vi "PSTR-Show PSTHs.vi"(0 "Data":T1, 5 "XYGraph":refnum<vi>, 7 "Freq":u16, 9 "Separation":dbl, 11 "Show fits":bool) -> ()   [LabVIEW 2020]
uses:
  Typedefs/PSTR-Data.ctl
  Typedefs/PSTR-Model Fit.ctl
  Typedefs/PSTR-Fit Parameters.ctl
  epl-vi-lib/Utility VIs/Math VIs/LinSpace (x0-dx-npts).vi
panel:
  # "NF x NL x 2 x Npts"
  # "NF x NL x Npts"
  # "NF x NL"
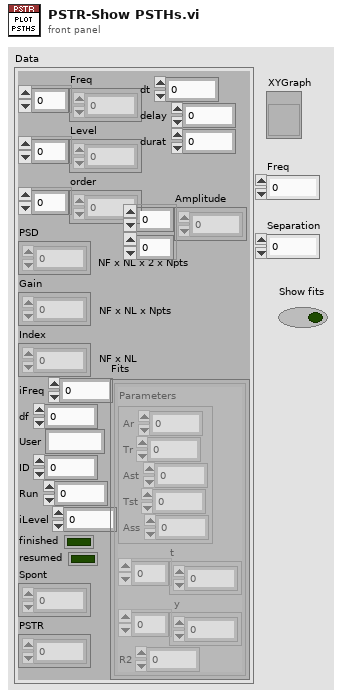
[diagram p1: front panel]
types:
  T1 = typedef "PSTR-Data.ctl" = cluster{"Freq":dbl[], "Level":dbl[], "order":i32[], "PSD":dbl[][][][], "Gain":dbl[][][], "Index":dbl[][], "iFreq":i32, "df":dbl, "User":string, "ID":i32, "Run":i32, "iLevel":i32, "finished":bool, "resumed":bool, "Spont":dbl[][], "PSTR":dbl[][][], "dt":dbl, "delay":dbl, "durat":dbl, "Fits":T2[][], "Amplitude":dbl[][]}
  T2 = typedef "PSTR-Model Fit.ctl" = cluster{"Parameters":T3, "t":dbl[], "y":dbl[], "R2":dbl}
  T3 = typedef "PSTR-Fit Parameters.ctl" = cluster{"Ar":dbl, "Tr":dbl, "Ast":dbl, "Tst":dbl, "Ass":dbl}
  T4 = enum16{"User", "Prism", "Kelly", "Dark2", "Sequential", "Hue"}
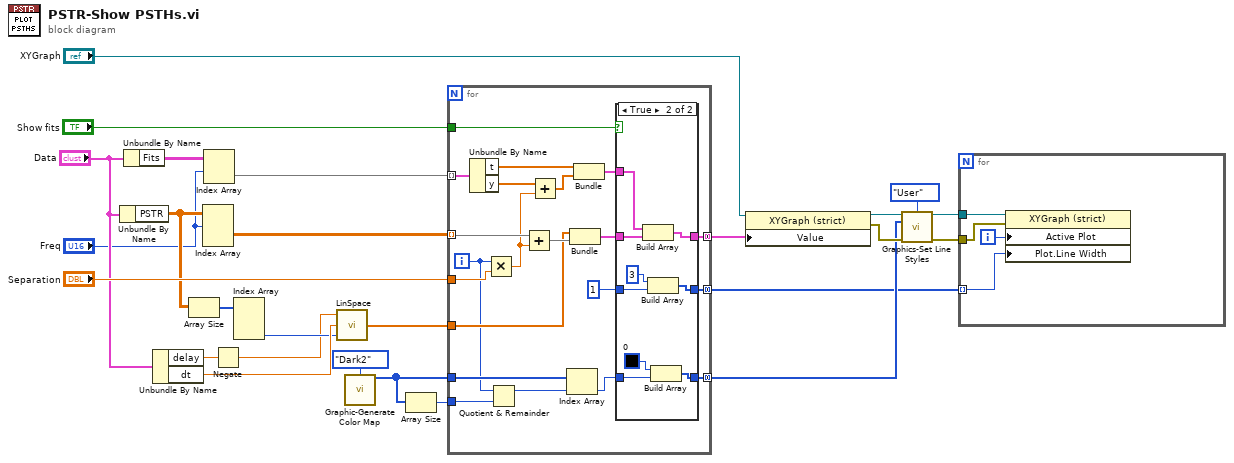
[diagram p0: block diagram]
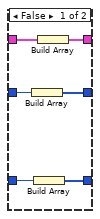
[diagram p2: hidden frame]
diagram:
  n1 = Unbundle By Name("Data") -> ("PSTR"=w21:dbl[][][])
  n2 = Unbundle By Name("Data") -> ("Fits"=w14:T2[][])
  n3 = Unbundle By Name("Data") -> ("delay"=w17:dbl, "dt"=w19:dbl)
  n4 = Array Size(array=w21) -> (size(s)=w20:i32[])
  n5 = Index Array(array=w21, index (dim 0)="Freq") -> (element=w4:dbl[][])  [unwired: 2 in]
  n6 = Index Array(array=w14, index (row)="Freq") -> (element=w5:T2[])  [unwired: 1 in]
  n7 = Negate(x=w17) -> (-x=w1:dbl)
  n8 = Index Array(array=w20) -> (element #3=w6:i32)  [unwired: 3 in, 2 out]
  n9 = call-poly "LinSpace.vi"("npts"=w6, "dx"=w19, "x0"=w1) -> ("Array"=w18:dbl[])  [unwired: 1 in, 1 out]
  n10 = call "Graphic-Generate Color Map.vi"("Map"=T4."Dark2") -> ("Colors"=w3:u32[])  [unwired: 14 in]
  n11 = Array Size(array=w3) -> (size(s)=w2:i32)
  n12 = for {
    tunnel: w4 -> [w47] mode=indexing
    tunnel: "Separation" -> [w46]
    tunnel: w18 -> [w44]
    tunnel: [w42] -> w16 mode=concatenating
    tunnel: w5 -> [w40] mode=indexing
    tunnel: "Show fits" -> [w43]
    tunnel: w3 -> [w31]
    tunnel: [w37] -> w10 mode=concatenating
    tunnel: [w33] -> w7 mode=concatenating
    tunnel: w2 -> [w29]
    i -> [w30]
    n13 = Unbundle By Name(w40) -> ("t"=w27:dbl[], "y"=w39:dbl[])
    n14 = Multiply(x=w30, y=w46) -> (x*y=w35:dbl)
    n15 = Quotient & Remainder(x=w30, y=w29) -> (x-y*floor(x/y)=w28:i32)  [unwired: 1 out]
    n16 = Add(x=w47, y=w35) -> (x+y=w45:dbl[])
    n17 = Add(x=w39, y=w35) -> (x+y=w36:dbl[])
    n18 = Index Array(array=w31, index=w28) -> (element=w32:u32)
    n19 = Bundle("Array"=w44, w45) -> (w41:cluster{"Array":dbl[], dbl[]})  [unwired: 1 in]
    n20 = Bundle("t"=w27, w36) -> (w38:cluster{"t":dbl[], dbl[]})  [unwired: 1 in]
    n21 = case shown="True" w43 {
      tunnel: [w52 w61] -> w42
      tunnel: w41 -> [w53 w62]
      tunnel: w38 -> [_ w60]
      tunnel: w32 -> [w51 w59]
      tunnel: [w50 w57] -> w37
      tunnel: u8 1 ("Plot.Line Width") -> [w49 w56]
      tunnel: [w48 w55] -> w33
      frame False {
        n22 = Build Array(w49) -> (w48:u8[])
        n23 = Build Array(w51) -> (w50:u32[])
        n24 = Build Array(w53) -> (w52:cluster{"Array":dbl[], dbl[]}[])
      }
      frame True {
        n25 = Build Array(w60, w62) -> (w61:cluster{"Array":dbl[], dbl[]}[])
        n26 = Build Array(u8 3 ("Plot.Line Width"), w56) -> (w55:u8[])
        n27 = Build Array(u32 0, w59) -> (w57:u32[])
      }
    }
  }
  n28 = property class="XYGraph (strict)"(reference="XYGraph", "Value"=w16) -> (reference out=w24:refnum<vi>, error out=w25:errorcluster)  [unwired: 1 in]
  n29 = call "Graphics-Set Line Styles.vi"("XY Graph"=w24, "Map"=enum16{"User", "Prism", "Kelly", "Dark2"}."User", "Colors"=w10, "error in (no error)"=w25) -> ("XY Graph out"=w9:refnum<vi>, "error out"=w8:errorcluster)  [unwired: 10 in]
  n30 = for {
    tunnel: w9 -> [w66]
    tunnel: w8 -> [w65]
    tunnel: w7 -> [w63] mode=indexing
    i -> [w64]
    n31 = property class="XYGraph (strict)"(reference=w66, error in=w65, "Active Plot"=w64, "Plot.Line Width"=w63) -> ()  [unwired: 2 out]
  }
